vi "Dispose.vi"(8 "error in (no error)":errorcluster, 11 "ConsoleOutput in":refnum<class "ConsoleOutput.lvclass">) -> (0 "error out":errorcluster)   [LabVIEW 2020, in "ConsoleOutput.lvclass"]
uses:
  ConsoleOutput.lvclass
  ConsoleOutput.lvclass/ConsoleOutput.ctl
  Lib/hse-logger.lvlib
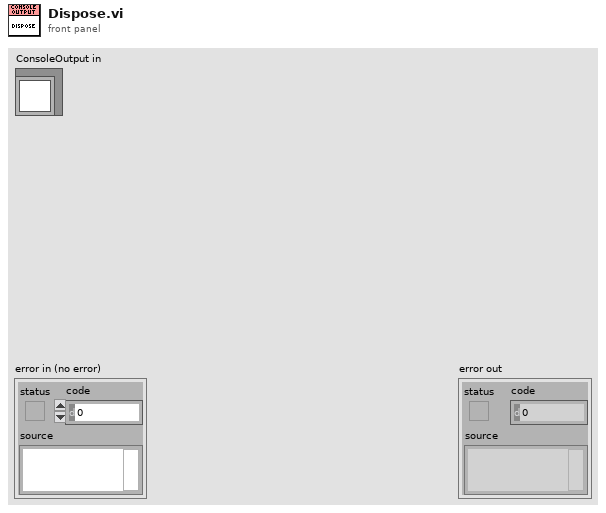
[diagram p1: front panel]
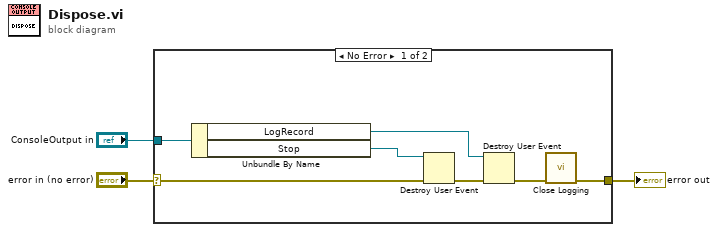
[diagram p0: block diagram]
diagram:
  n1 = case shown="No Error" "error in (no error)" {
    selector: "error in (no error)" -> [w4 w11]
    tunnel: [w5 w11] -> w2
    tunnel: "ConsoleOutput in" -> [w10 _]
    frame No Error {
      n2 = Unbundle By Name(w10) -> ("LogRecord"=w8:refnum<user-event>, "Stop"=w7:refnum<user-event>)
      n3 = Destroy User Event(user event=w7, error in=w4) -> (error out=w9:errorcluster)
      n4 = Destroy User Event(user event=w8, error in=w9) -> (error out=w6:errorcluster)
      n5 = call "Close Logging.vi"("error in"=w6) -> ("error out"=w5:errorcluster)  [unwired: 10 in]
    }
    frame Error {
    }
  }
  "error out" <- w2
